vi "Create_Trajectory_Value_Meters_To_Units.vi"(6 "Units Selector":T1, 11 "Meters":dbl) -> (3 "Units":dbl)   [LabVIEW 2019]
doc: "Convert given units to Meter"
uses:
  TrajCreateUnitsENUM.ctl
  <vilib>/Rock Robotics/WPI/ThirdParty/JAS_Junk/TrajLib/Trajectory_Library.lvlib
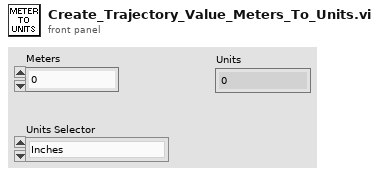
[diagram p1: front panel]
types:
  T1 = typedef "TrajCreateUnitsENUM.ctl" = enum16{"Inches", "Feet", "Centimeters", "Meters"}
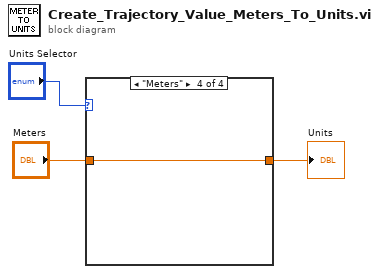
[diagram p0: block diagram]
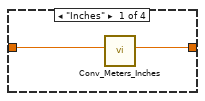
[diagram p2: hidden frame]
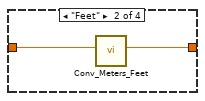
[diagram p3: hidden frame]
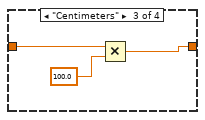
[diagram p4: hidden frame]
diagram:
  n1 = case shown="\"Meters\"" "Units Selector" {
    tunnel: [w4 w6 w8 w11] -> w3
    tunnel: "Meters" -> [w5 w7 w10 w11]
    frame "Inches" {
      n2 = call <vilib>:"Conv_Meters_Inches.vi"("Meters"=w5) -> ("Inches"=w4:dbl)  [unwired: 10 in]
    }
    frame "Feet" {
      n3 = call <vilib>:"Conv_Meters_Feet.vi"("Meters"=w7) -> ("Feet"=w6:dbl)  [unwired: 10 in]
    }
    frame "Centimeters" {
      n4 = Multiply(x=w10, y=100.0) -> (x*y=w8:dbl)
    }
    frame "Meters" {
    }
  }
  "Units" <- w3
